vi "Elevator Control Loop.vi"() -> ()   [LabVIEW 2014, in "Elevator System.lvlib"]
uses:
  Elevator System.lvlib
  <vilib>/Rock Robotics/WPI/MotorControl/WPI_MotorControlDeviceRef.ctl
  <vilib>/Rock Robotics/WPI/MotorControl/WPI_MotorControlType.ctl
  <vilib>/Rock Robotics/SystemInterfaces/Typedef/FPGA_TypedefDigitalModule.ctl
  <vilib>/Rock Robotics/SystemInterfaces/DIO/FPGA_DIOPWMChannel.ctl
  <vilib>/Rock Robotics/WPI/PWM/WPI_PWMDeadband.ctl
  <vilib>/Rock Robotics/WPI/CAN/Jaguar/SubVIs/WPI_CANJaguar_ControlMode.ctl
  <vilib>/Rock Robotics/WPI/CAN/TalonSRX/WPI_CANTalonSRX_APIControlMode.ctl
  <vilib>/Rock Robotics/WPI/PWM/WPI_PWMTransform_ConPane.ctl
  Public/Sensors Global.vi
  <vilib>/addons/control/pid/pid.llb/PID (DBL).vi
  <vilib>/addons/control/pid/NI_PID_pid.lvlib
panel:
  out "Plant Input":dbl(graph)
  in  "output range":cluster{"output high":dbl, "output low":dbl}={"output high"=100.0, "output low"=-1.0} {"output low" format="%.2f"; "output high" format="%.2f"}
  in  "PID gains":T1={"proportional gain (Kc)"=11.9, "integral time (Ti, min)"=0.004, "derivative time (Td, min)"=0.0} {"derivative time (Td, min)" format="%.3f"; "integral time (Ti, min)" format="%.3f"; "proportional gain (Kc)" format="%.3f"}
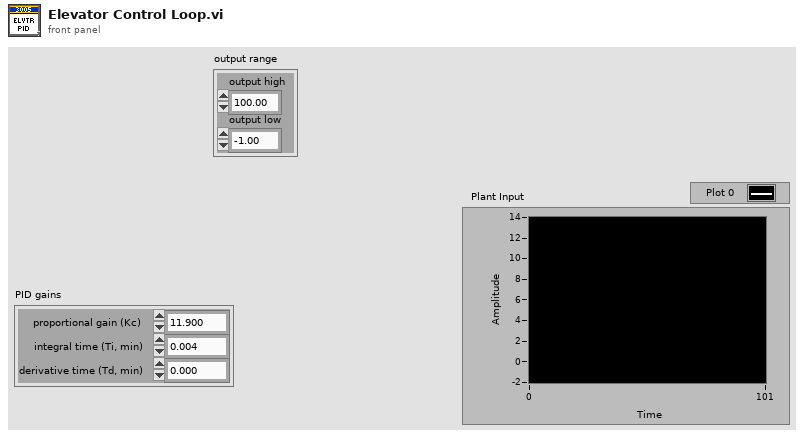
[diagram p1: front panel]
types:
  T1 = cluster{"proportional gain (Kc)":dbl, "integral time (Ti, min)":dbl, "derivative time (Td, min)":dbl}
  T2 = typedef "WPI_MotorControlDeviceRef.ctl" = cluster{"DeviceStatus":errorcluster, "Type":T3, "PWM":cluster{"Controller":T4, "PWM Channel":T5, "DeadBand":T6}, "CAN":cluster{"Device Number":u8, "Control Mode":T7, "Semaphore":T8, "Max Vout":dbl, "TalonSRX Control Mode":T9}, "Invert":bool, "TransformRef":T10, "InvTransformRef":T10}
  T3 = typedef "WPI_MotorControlType.ctl" = enum16{"PWM", "CAN", "CANTalonSRX"}
  T4 = typedef "FPGA_TypedefDigitalModule.ctl" = enum16{"Controller 1"}
  T5 = typedef "FPGA_DIOPWMChannel.ctl" = enum8{"PWM 0", "PWM 1", "PWM 2", "PWM 3", "PWM 4", "PWM 5", "PWM 6", "PWM 7", "PWM 8", "PWM 9", "PWM MXP 0", "PWM MXP 1", "PWM MXP 2", "PWM MXP 3", "PWM MXP 4", "PWM MXP 5", "PWM MXP 6", "PWM MXP 7", "PWM MXP 8", "PWM MXP 9", "Invalid"}
  T6 = typedef "WPI_PWMDeadband.ctl" = cluster{"Name":string, "maxPositivePwm":i32, "minPositivePwm":i32, "centerPwm":i32, "maxNegativePwm":i32, "minNegativePwm":i32, "angularRange":u16}
  T7 = typedef "WPI_CANJaguar_ControlMode.ctl" = enum8{"Percent VBus", "Current", "Speed", "Position", "Voltage"}
  T8 = typedef "Semaphore RefNum" = refnum<k1>
  T9 = typedef "WPI_CANTalonSRX_APIControlMode.ctl" = enum8{"Percent VBus", "Speed", "Position", "Slave", "Unchanged / Invalid"}
  T10 = typedef "WPI_PWMTransform_ConPane.ctl" = refnum<vi>
  T11 = cluster{"Setpoint":dbl, "notifier out":refnum<notifier>, "Output":dbl, "DriveMotor":T2}
  T12 = cluster{"static gain":dbl, "lag (s)":dbl, "deadtime (s)":dbl, "load":dbl, "deadband":dbl, "sensor noise":dbl, "initial PV":dbl, "plant noise":dbl}
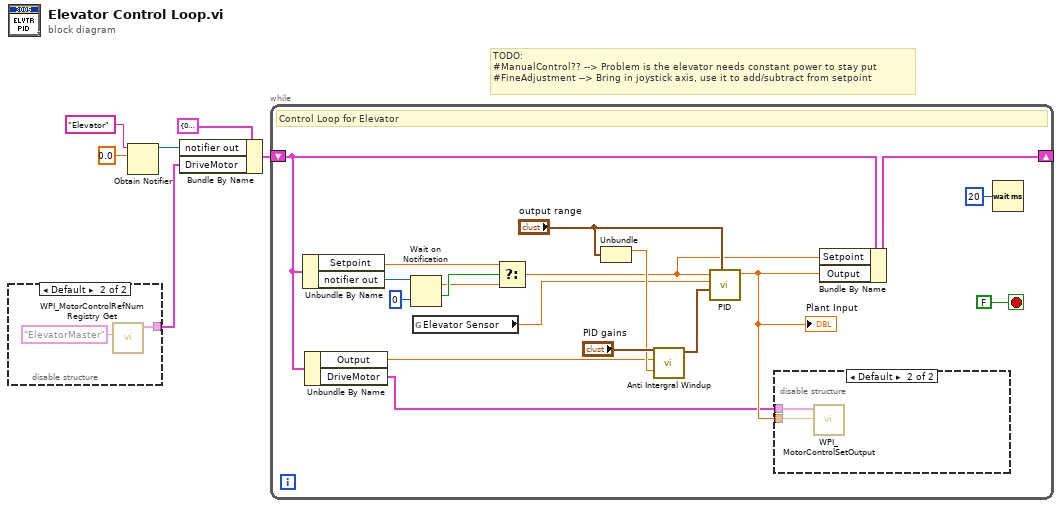
[diagram p0: block diagram]
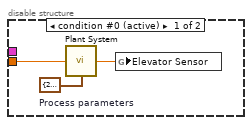
[diagram p3: hidden frame]
diagram:
  # "TODO:\n#ManualControl?? --> Problem is the elevator needs constant power to stay put\n#FineAdjustment --> Bring in joystick axis, use it to add/subtract from setpoint"
  n1 = disable-structure shown="Default" {
    disable-tunnel: [_ w8] -> w1
    frame condition #0 (active) {
    }
    frame condition #1 {
      n2 = call <vilib>:"WPI_MotorControlRefNum Registry Get.vi"("refnum name"="ElevatorMaster") -> ("MotorControlDevRef"=w8:T2)  [unwired: 9 in, 1 out]
    }
  }
  n3 = Obtain Notifier(name (unnamed)="Elevator", notification data type=0.0 ("Setpoint")) -> (notifier out=w4:refnum<notifier>)  [unwired: 2 in, 2 out]
  n4 = Bundle By Name(cluster=T11 {"Setpoint"=0.0, "notifier out"=refnum, "Output"=0.0, "DriveMotor"={"DeviceStatus"={"status"=FALSE, "code"=0, "source"=""}, "Type"=enum."PWM", "PWM"={"Controller"=enum."Controller 1", "PWM Channel"=enum."Invalid", "DeadBand"={"Name"="", "maxPositivePwm"=0, "minPositivePwm"=0, "centerPwm"=0, "maxNegativePwm"=0, "minNegativePwm"=0, "angularRange"=0}}, "CAN"={"Device Number"=0, "Control Mode"=enum."Percent VBus", "Semaphore"=refnum, "Max Vout"=12.0, "TalonSRX Control Mode"=enum."Percent VBus"}, "Invert"=FALSE, "TransformRef"=refnum, "InvTransformRef"=refnum}}, "notifier out"=w4, "DriveMotor"=w1) -> (w5:T11)
  n5 = while {
    shift-right: [w18] -> _
    shift-left: w5 -> [w17]
    stop <- FALSE stop-if-true
    # "Control Loop for Elevator"
    n6 = Unbundle By Name(w17) -> ("Setpoint"=w23:dbl, "notifier out"=w25:refnum<notifier>)
    n7 = Unbundle By Name(w17) -> ("Output"=w16:dbl, "DriveMotor"=w9:T2)
    n8 = Wait on Notification(notifier=w25, timeout in ms (-1)=0) -> (notification=w10:dbl, timed out?=w24:bool)  [unwired: 2 in, 2 out]
    n9 = global read "Sensors Global.vi" "Elevator Sensor"() -> (w15:dbl)
    n10 = Select(t=w23, s=w24, f=w10) -> (s? t:f=w13:dbl)
    n11 = Unbundle("output range") -> ("output high"=w19:dbl)  [unwired: 1 out]
    n12 = call "Anti Intergral Windup.vi"("|Limit|"=w19, "MV"=w16, "PID gains"="PID gains") -> ("PID gains"=w21:T1)  [unwired: 8 in]
    n13 = call-poly <vilib>:"PID.vi"("output range"="output range", "PID gains"=w21, "process variable"=w15, "setpoint"=w13) -> ("output"=w14:dbl)  [unwired: 6 in, 1 out]
    "Plant Input" <- w14
    n14 = disable-structure shown="Default" {
      disable-tunnel: w14 -> [w28 w31]
      disable-tunnel: w9 -> [_ w30]
      frame condition #0 (active) {
        w29 = T12 {"static gain"=2.5, "lag (s)"=2.5, "deadtime (s)"=0.01, "load"=30.0, "deadband"=0.0, "sensor noise"=0.0, "initial PV"=6.0, "plant noise"=0.0}  # Process parameters
        n15 = call "Plant System.vi"("Plant Input"=w28, "process parameters"=w29) -> ("Plant Output"=w27:dbl)  [unwired: 13 in]
        n16 = global write "Sensors Global.vi" "Elevator Sensor"(w27) -> ()
      }
      frame condition #1 {
        n17 = call <vilib>:"WPI_MotorControlSetOutput.vi"("Output"=w31, "MotorControlDevRef"=w30) -> ()  [unwired: 7 in, 3 out]
      }
    }
    n18 = Bundle By Name(cluster=w17, "Setpoint"=w13, "Output"=w14) -> (w18:T11)
    n19 = Wait (ms)(milliseconds to wait=u32 20) -> ()  [unwired: 1 out]
  }
